vi "Write Configuration Settings File.vi"() -> ()   [LabVIEW 2017]
doc: "Illustrates how to create and write a configuration settings file.\n\nInstructions:\nEnter values in the controls on the front panel then click on the Run Arrow.\nTo read the file, run Read Configuration Settings File.vi located in the file\\config.llb."
uses:
  Configuration Data.ctl
  Car Wash System Globals.vi
  <vilib>/Utility/config.llb/Write Key (U32).vi
  <vilib>/Utility/config.llb/NI_LVConfig.lvlib
panel:
  in  "Cluster":T1
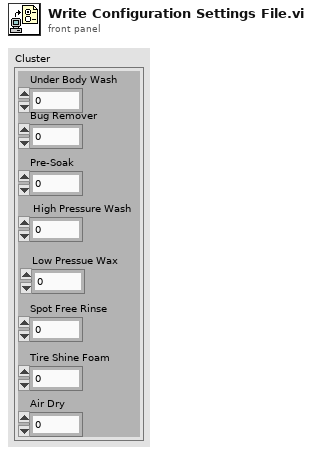
[diagram p1: front panel]
types:
  T1 = typedef "Configuration Data.ctl" = cluster{"Under Body Wash ":u32, "Bug Remover":u32, "Pre-Soak":u32, " High Pressure Wash":u32, "Low Pressue Wax ":u32, "Spot Free Rinse ":u32, "Tire Shine Foam":u32, "Air Dry ":u32}
  T2 = typedef "NI_LVConfig.lvlib/Config Data RefNum.ctl" = refnum<k1>
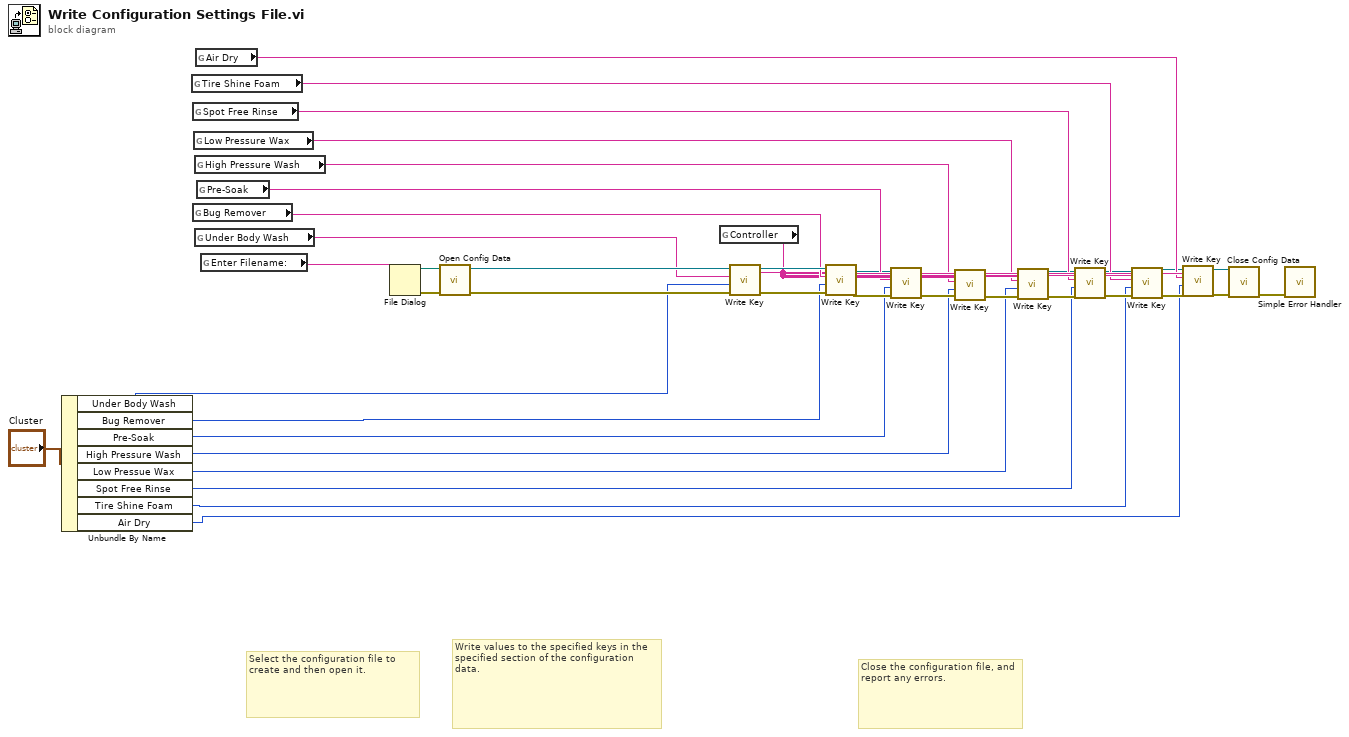
[diagram p0: block diagram]
diagram:
  # "Close the configuration file, and report any errors."
  # "Write values to the specified keys in the specified section of the configuration data."
  # "Select the configuration file to create and then open it."
  n1 = Unbundle By Name("Cluster") -> ("Under Body Wash"=w8:u32, "Bug Remover"=w7:u32, "Pre-Soak"=w6:u32, "High Pressure Wash"=w5:u32, "Low Pressue Wax"=w4:u32, "Spot Free Rinse"=w3:u32, "Tire Shine Foam"=w2:u32, "Air Dry"=w1:u32)
  n2 = global read "Car Wash System Globals.vi" "Tire Shine Foam"() -> (w18:string)
  n3 = global read "Car Wash System Globals.vi" "Spot Free Rinse"() -> (w19:string)
  n4 = global read "Car Wash System Globals.vi" "Bug Remover"() -> (w24:string)
  n5 = global read "Car Wash System Globals.vi" "Low Pressure Wax"() -> (w20:string)
  n6 = global read "Car Wash System Globals.vi" "High Pressure Wash"() -> (w21:string)
  n7 = global read "Car Wash System Globals.vi" "Under Body Wash"() -> (w25:string)
  n8 = global read "Car Wash System Globals.vi" "Air Dry"() -> (w17:string)
  n9 = global read "Car Wash System Globals.vi" "Pre-Soak"() -> (w22:string)
  n10 = global read "Car Wash System Globals.vi" "Enter Filename:"() -> (w26:string)
  n11 = File Dialog(7:w26) -> (0:w38:errorcluster, 3:w40:path)  [unwired: 1 in, 7 out]
  n12 = call <vilib>:"Open Config Data.vi"("error in (no error)"=w38, "configuration file path"=w40) -> ("error out"=w34:errorcluster, "refnum"=w35:T2)  [unwired: 1 in, 7 out]
  n13 = global read "Car Wash System Globals.vi" "Controller"() -> (w23:string)
  n14 = call-poly <vilib>:"Write Key.vi"("section"=w23, "error in (no error)"=w34, "value"=w8, "key"=w25, "refnum"=w35) -> ("error out"=w37:errorcluster, "refnum out"=w36:T2)  [unwired: 4 in, 1 out]
  n15 = call-poly <vilib>:"Write Key.vi"("section"=w23, "error in (no error)"=w37, "value"=w7, "key"=w24, "refnum"=w36) -> ("error out"=w33:errorcluster, "refnum out"=w11:T2)  [unwired: 4 in, 1 out]
  n16 = call-poly <vilib>:"Write Key.vi"("section"=w23, "error in (no error)"=w33, "value"=w6, "key"=w22, "refnum"=w11) -> ("error out"=w32:errorcluster, "refnum out"=w12:T2)  [unwired: 4 in, 1 out]
  n17 = call-poly <vilib>:"Write Key.vi"("section"=w23, "error in (no error)"=w32, "value"=w5, "key"=w21, "refnum"=w12) -> ("error out"=w31:errorcluster, "refnum out"=w13:T2)  [unwired: 4 in, 1 out]
  n18 = call-poly <vilib>:"Write Key.vi"("section"=w23, "error in (no error)"=w31, "value"=w4, "key"=w20, "refnum"=w13) -> ("error out"=w30:errorcluster, "refnum out"=w14:T2)  [unwired: 4 in, 1 out]
  n19 = call-poly <vilib>:"Write Key.vi"("section"=w23, "error in (no error)"=w30, "value"=w3, "key"=w19, "refnum"=w14) -> ("error out"=w29:errorcluster, "refnum out"=w15:T2)  [unwired: 4 in, 1 out]
  n20 = call-poly <vilib>:"Write Key.vi"("section"=w23, "error in (no error)"=w29, "value"=w2, "key"=w18, "refnum"=w15) -> ("error out"=w28:errorcluster, "refnum out"=w16:T2)  [unwired: 4 in, 1 out]
  n21 = call-poly <vilib>:"Write Key.vi"("section"=w23, "error in (no error)"=w28, "value"=w1, "key"=w17, "refnum"=w16) -> ("error out"=w27:errorcluster, "refnum out"=w10:T2)  [unwired: 4 in, 1 out]
  n22 = call <vilib>:"Close Config Data.vi"("error in (no error)"=w27, "refnum"=w10) -> ("error out"=w39:errorcluster)  [unwired: 1 in, 8 out]
  n23 = call <vilib>:"Simple Error Handler.vi"("error in (no error)"=w39) -> ()  [unwired: 1 in, 8 out]
